vi "params.From JSON Tree.vi"(8 "error in (no error)":errorcluster, 10 "JSON Value in":variant, 11 "params in":refnum<class "params.lvclass">) -> (0 "error out":errorcluster, 3 "params in":refnum<class "params.lvclass">)   [LabVIEW 2020, in "JSON-RPC Lib.lvlib" / "params.lvclass"]
uses:
  params.lvclass
  params.lvclass/params.ctl
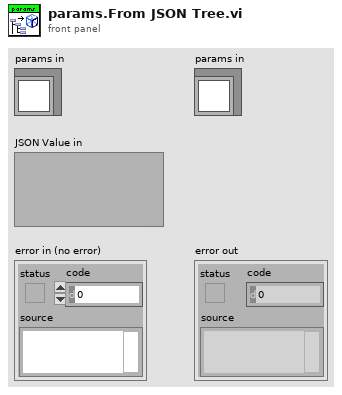
[diagram p1: front panel]
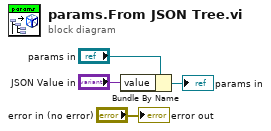
[diagram p0: block diagram]
diagram:
  n1 = Bundle By Name(cluster="params in", "value"="JSON Value in") -> (→"params in":refnum<class "params.lvclass">)
  "error out" <- "error in (no error)"
